vi "clearPropertyValue.vi"(8 "error in (no error)":errorcluster, 10 "Property Name in":string, 11 "IPropertyObject in":refnum<class "IPropertyObject.lvclass">) -> (0 "error out":errorcluster, 3 "IPropertyObject out":refnum<class "IPropertyObject.lvclass">)   [LabVIEW 2022 SP3, in "openDAQ.lvlib" / "IBaseObject.lvlib" / "IPropertyObject.lvlib" / "IPropertyObject.lvclass"]
uses:
  <instrlib>/openDAQ/Public/Classes/IPropertyObject/IPropertyObject.lvclass
  <instrlib>/openDAQ/Public/Classes/IPropertyObject/IPropertyObject.lvclass/IPropertyObject.ctl
  <instrlib>/openDAQ/Public/Classes/daqCoreTypes/IString/IString.lvclass
  <instrlib>/openDAQ/Binaries/Windows/x86/copendaq32.dll
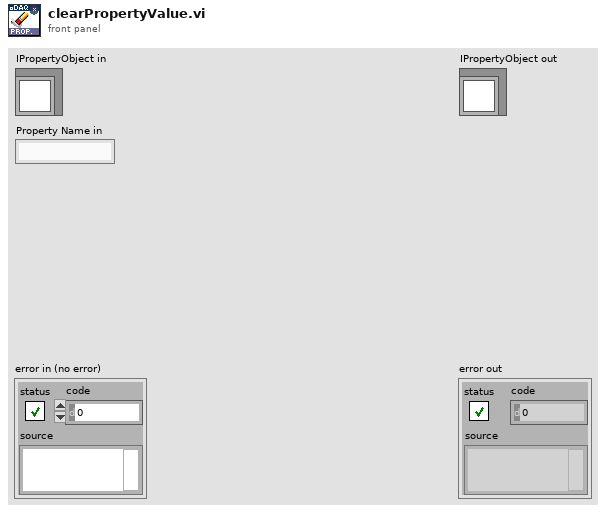
[diagram p1: front panel]
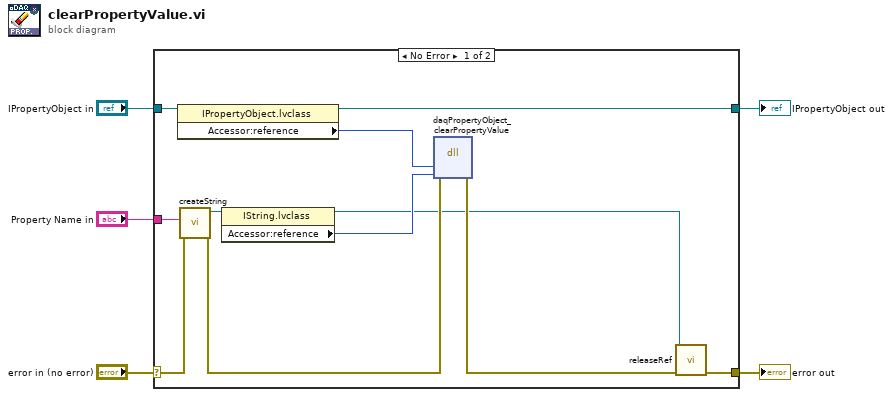
[diagram p0: block diagram]
diagram:
  n1 = case shown="No Error" "error in (no error)" {
    selector: "error in (no error)" -> [w13 w18]
    tunnel: [w8 w18] -> w4
    tunnel: [w14 w17] -> w2
    tunnel: "IPropertyObject in" -> [w16 w17]
    tunnel: "Property Name in" -> [w11 _]
    frame No Error {
      n2 = property class="IPropertyObject.lvclass"(reference=w16) -> (reference out=w14:refnum<class "IPropertyObject.lvclass">, "Accessor:reference"=w15:i64)  [unwired: 1 in, 1 out]
      n3 = call <instrlib>:"createString.vi"("error in (no error)"=w13, "String"=w11) -> ("error out"=w12:errorcluster, "IString out"=w10:refnum<class "IString.lvclass">)  [unwired: 8 in]
      n4 = property class="IString.lvclass"(reference=w10) -> (reference out=w6:refnum<class "IString.lvclass">, "Accessor:reference"=w9:i64)  [unwired: 1 in, 1 out]
      n5 = dll-call lib="C:/Program Files (x86)/National Instruments/LabVIEW 2022/instr.lib/openDAQ/Binaries/Windows/x86/copendaq*.*" fn="daqPropertyObject_clearPropertyValue"(error in=w12, "propertyObject"=w15, "name"=w9) -> (error out=w7:errorcluster)  [unwired: 5 in, 1 out]
      n6 = call-dynamic "releaseRef.vi"("error in (no error)"=w7, "IBaseObject in"=w6) -> ("error out"=w8:errorcluster)  [unwired: 9 in]
    }
    frame Error {
    }
  }
  "error out" <- w4
  "IPropertyObject out" <- w2
